vi "Examen.vi"() -> ()   [LabVIEW 2017]
uses:
  C:/Users/h16034903/Downloads/Masure_Henry_projet.llb/Variable globale 1.vi
panel:
  out "cluster de sortie 2":T1
  out "Fréquence échantillonnage":dbl
  in  "Enregistrer données":bool
  in  "Ajouter un commentaire":bool
  in  "Commentaire":string
  out "Date examen":timestamp
  out "Nom":string
  out "Prénom":string
  out "Tracés de l'ECG":dbl[][](graph)
  out "Mémorisation de données":dbl[][](array[numeric])
  in  "Stop":bool
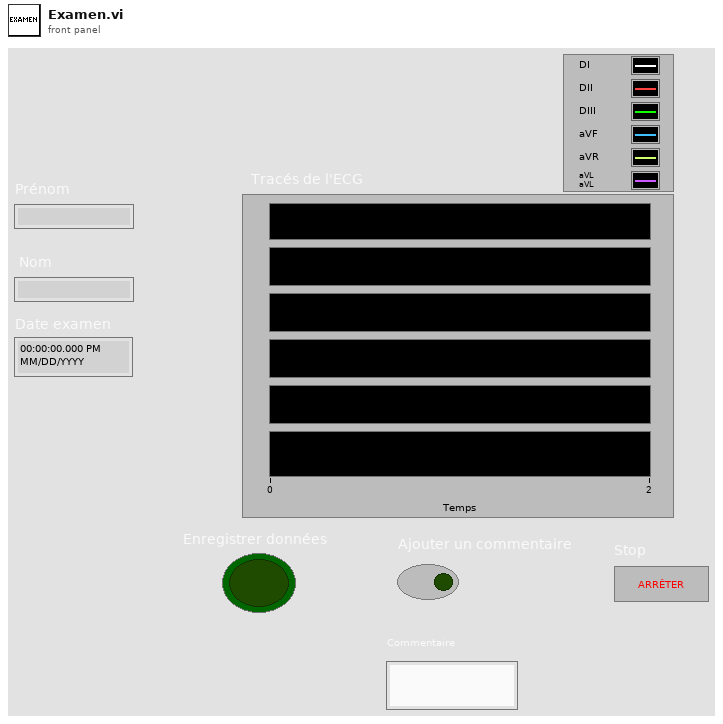
[diagram p1: front panel]
types:
  T1 = cluster{"frequence echantillonage":dbl, "ECG filtré\n":dbl[][], string[], "Nom":string, "Prénom":string, "Date de l'examen":timestamp, i32[]}
  T2 = cluster{"frequence echantillonage":dbl, dbl[][], string[], "Nom":string, "Prénom":string, "Date de l'examen":timestamp, i32[]}
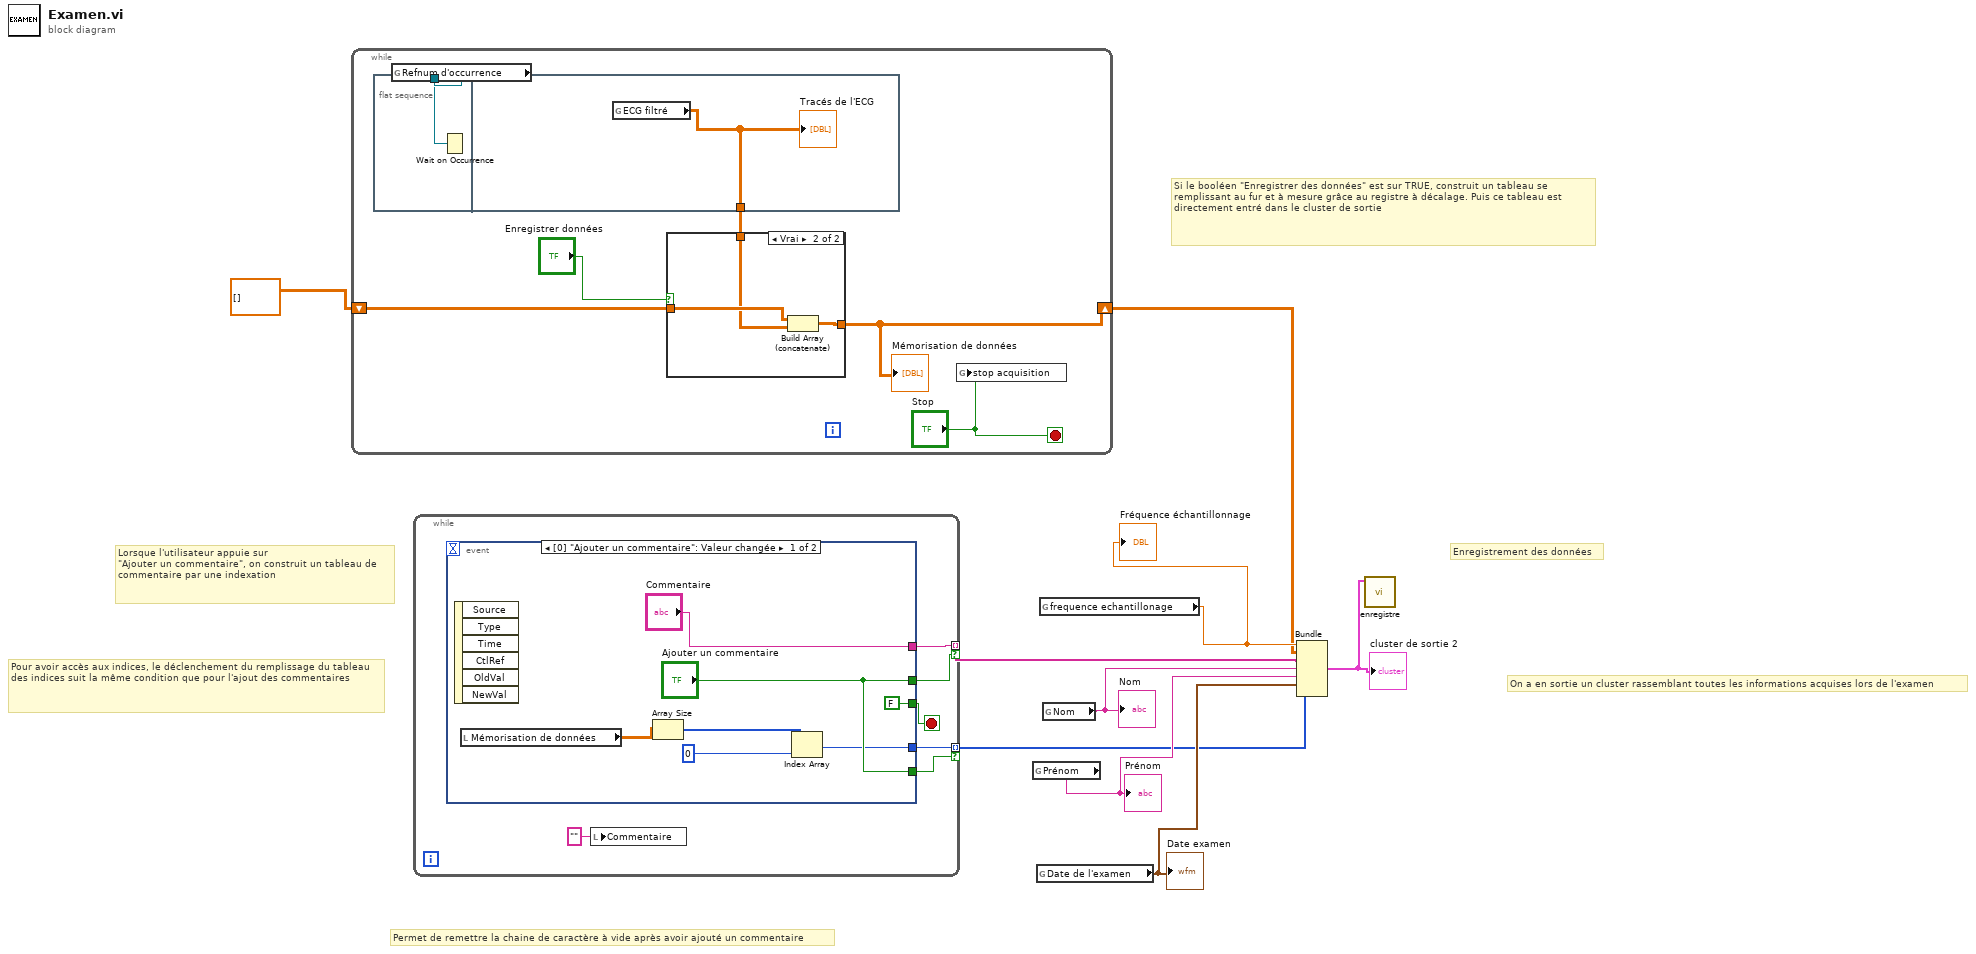
[diagram p0: block diagram]
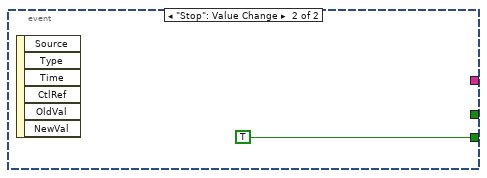
[diagram p2: hidden frame]
diagram:
  # "On a en sortie un cluster rassemblant toutes les informations acquises lors de l'examen"
  # "Pour avoir accès aux indices, le déclenchement du remplissage du tableau des indices suit la même condition que pour l'ajout des commentaires"
  # "Lorsque l'utilisateur appuie sur\n\"Ajouter un commentaire\", on construit un tableau de commentaire par une indexation"
  # "Si le booléen \"Enregistrer des données\" est sur TRUE, construit un tableau se remplissant au fur et à mesure grâce au registre à décalage. Puis ce tableau est directement entré dans le cluster de sortie"
  # "Permet de remettre la chaine de caractère à vide après avoir ajouté un commentaire"
  # "Enregistrement des données"
  n1 = while {
    shift-right: [w10] -> w2
    shift-left: dbl[][] [] -> [w12]
    stop <- "Stop" stop-if-true
    n2 = flat-sequence {
      tunnel: w15 -> [w20]
      tunnel: [w21] -> w11
      frame #0 {
        n3 = Wait on Occurrence(2:w20) -> ()  [unwired: 2 in, 1 out]
      }
      frame #1 {
        n4 = global read "Variable globale 1.vi" "ECG filtré"() -> (w21:dbl[][])
        "Tracés de l'ECG" <- w21
      }
    }
    n5 = global read "Variable globale 1.vi" "Refnum d'occurrence"() -> (w15:refnum<k4>)
    n6 = case shown="Vrai" "Enregistrer données" {
      tunnel: w12 -> [w16 w19]
      tunnel: [w16 w17] -> w10
      tunnel: w11 -> [_ w18]
      frame False {
      }
      frame True {
        n7 = Build Array (concatenate)(w19, w18) -> (w17:dbl[][])
      }
    }
    "Mémorisation de données" <- w10
    n8 = global write "Variable globale 1.vi" "stop acquisition"("Stop") -> ()
  }
  n9 = while {
    tunnel: [w26] -> w8 mode=indexing if=w27
    tunnel: [w22] -> w4 mode=indexing if=w23
    stop <- w25 stop-if-true
    n10 = event shown="[0] \"Ajouter un commentaire\": Valeur changée" {
      selector: _ -> [_ _]
      dyn-events: _ -> [_ _]
      timeout: _ -> [_ _]
      tunnel: ["Ajouter un commentaire" _] -> w27
      tunnel: ["Commentaire" _] -> w26
      tunnel: [FALSE TRUE] -> w25
      tunnel: ["Ajouter un commentaire" _] -> w23
      tunnel: [w29 _] -> w22
      event "Ajouter un commentaire": Value Change {
        n11 = event-data() -> ()  [unwired: 1 in, 6 out]
        n12 = local read "Mémorisation de données"() -> (w28:dbl[][])
        n13 = Array Size(array=w28) -> (size(s)=w33:i32[])
        n14 = Index Array(array=w33, index=0 ("indice")) -> (element=w29:i32)
      }
      event "Stop": Value Change {
        n15 = event-data() -> ()  [unwired: 1 in, 6 out]
      }
    }
    n16 = local write "Commentaire"("" ("Commentaire")) -> ()
  }
  n17 = global read "Variable globale 1.vi" "Prénom"() -> (w6:string)
  "Prénom" <- w6
  n18 = global read "Variable globale 1.vi" "Date de l'examen"() -> (w5:timestamp)
  "Date examen" <- w5
  n19 = global read "Variable globale 1.vi" "frequence echantillonage"() -> (w9:dbl)
  "Fréquence échantillonnage" <- w9
  n20 = global read "Variable globale 1.vi" "Nom"() -> (w7:string)
  "Nom" <- w7
  n21 = Bundle("frequence echantillonage"=w9, w2, w8, "Nom"=w7, "Prénom"=w6, "Date de l'examen"=w5, w4) -> (w1:T2)  [unwired: 1 in]
  "cluster de sortie 2" <- w1
  n22 = call "enregistre.vi"("cluster de sortie 2"=w1) -> ()  [unwired: 11 in]
